vi "Print Number.vi"(8 "error in (no error)":errorcluster, 9 "Input":string, 11 "VISA resource name":refnum<visa-resource-name>) -> (0 "error out":errorcluster, 1 "Output":string, 3 "VISA resource name out":refnum<visa-resource-name>, 4 "Command String":string)   [LabVIEW 2017, in "Keithley 2600 Series.lvlib"]
doc: "This VI instructs the instrument to print the contents of the test script variable or value named by Input, to the instrument's output data queue. The returned data will be formatted according to the instrument format attributes.\n\nSee Also: format.data, format.asciiprecision, format.byteorder\n\n<b>Functions and Attributes Used</b>\nprintnumber()"
uses:
  Keithley 2600 Series.lvlib
  Private/GlobalVariables.vi
panel:
  # "(c) 2008 Keithley Instruments, Inc.  ALL RIGHTS RESERVED."
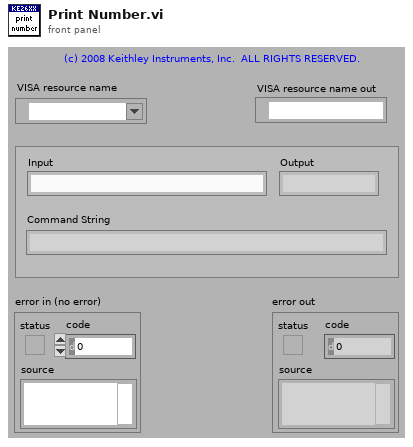
[diagram p1: front panel]
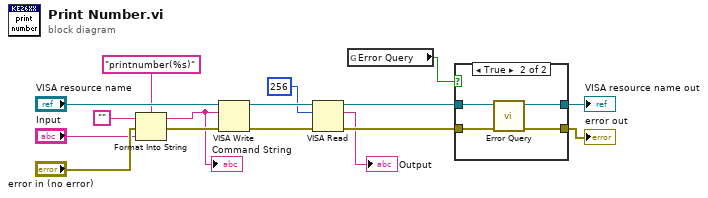
[diagram p0: block diagram]
diagram:
  n1 = Format Into String(format string="printnumber(%s)" ("initial string"), initial string="", error in="error in (no error)", "Input") -> (resulting string=w10:string, error out=w12:errorcluster)
  "Command String" <- w10
  n2 = VISA Write(VISA resource name="VISA resource name", write buffer=w10, error in (no error)=w12) -> (VISA resource name out=w13:refnum<visa-resource-name>, error out=w3:errorcluster)  [unwired: 1 out]
  n3 = VISA Read(VISA resource name=w13, byte count=u32 256, error in (no error)=w3) -> (VISA resource name out=w6:refnum<visa-resource-name>, read buffer=→"Output":string, error out=w5:errorcluster)  [unwired: 1 out]
  n4 = global read "GlobalVariables.vi" "Error Query"() -> (w7:bool)
  n5 = case shown="True" w7 {
    tunnel: w6 -> [w18 w22]
    tunnel: w5 -> [w17 w21]
    tunnel: [w18 w20] -> w4
    tunnel: [w17 w19] -> w16
    frame False {
    }
    frame True {
      n6 = call "Error Query.vi"("error in (no error)"=w21, "VISA resource name"=w22) -> ("error out"=w19:errorcluster, "VISA resource name out"=w20:refnum<visa-resource-name>)  [unwired: 8 out]
    }
  }
  "error out" <- w16
  "VISA resource name out" <- w4
